vi "Write Analysis Data.vi"(8 "error in (no error)":errorcluster, 10 "Analysis Data":T1, 11 "Optical Spectrum Analyzer in":refnum<class "Optical Spectrum Analyzer.lvclass">) -> (0 "error out":errorcluster, 3 "Optical Spectrum Analyzer out":refnum<class "Optical Spectrum Analyzer.lvclass">)   [LabVIEW 2018, in "Optical Spectrum Analyzer.lvlib" / "Optical Spectrum Analyzer.lvclass"]
uses:
  Optical Spectrum Analyzer.lvclass
  Custom Controls/Analysis Data.ctl
  Optical Spectrum Analyzer.lvclass/Optical Spectrum Analyzer.ctl
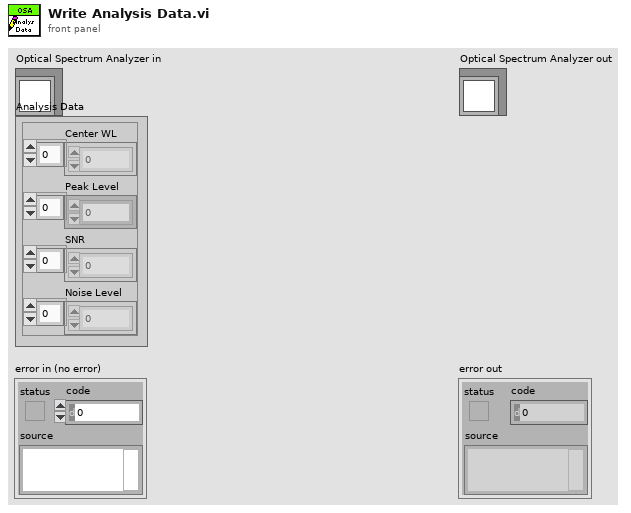
[diagram p1: front panel]
types:
  T1 = typedef "Optical Spectrum Analyzer.lvlib/Optical Spectrum Analyzer.lvclass/Analysis Data.ctl" = cluster{"Center WL":dbl[], "Peak Level":dbl[], "SNR":dbl[], "Noise Level":dbl[]}
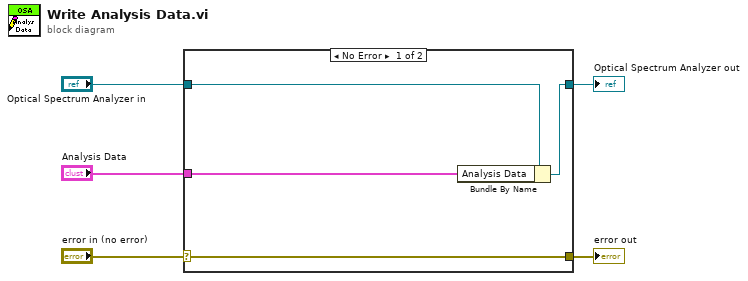
[diagram p0: block diagram]
diagram:
  n1 = case shown="No Error" "error in (no error)" {
    selector: "error in (no error)" -> [w9 w10]
    tunnel: [w9 w10] -> w4
    tunnel: [w7 w11] -> w2
    tunnel: "Optical Spectrum Analyzer in" -> [w8 w11]
    tunnel: "Analysis Data" -> [w6 _]
    frame No Error {
      n2 = Bundle By Name(cluster=w8, "Analysis Data"=w6) -> (w7:refnum<class "Optical Spectrum Analyzer.lvclass">)
    }
    frame Error {
    }
  }
  "error out" <- w4
  "Optical Spectrum Analyzer out" <- w2
